vi "反馈节点 3.vi"() -> ()   [LabVIEW 2023]
panel:
  out "i=":i32
  out "x+1":dbl
  out "Array":dbl[](array[numeric])
  # "反馈节点 3"
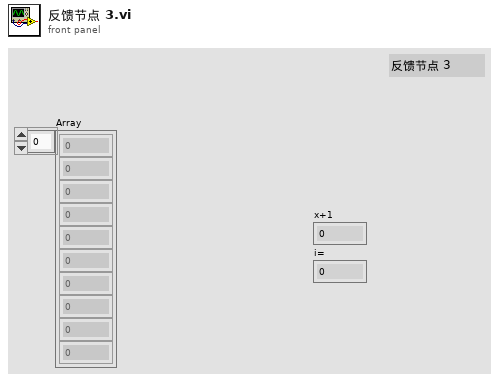
[diagram p1: front panel]
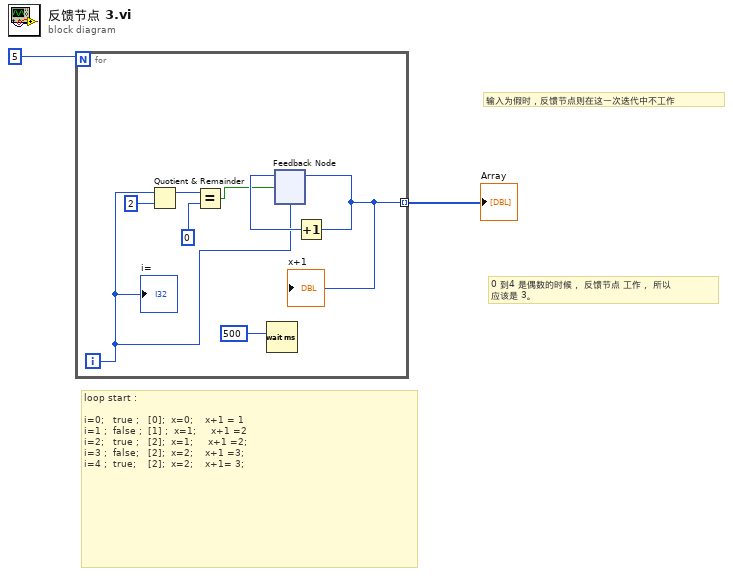
[diagram p0: block diagram]
diagram:
  # "0 到4 是偶数的时候， 反馈节点 工作， 所以 \n应该是 3。"
  # "loop start :\n\ni=0;   true ;   [0];  x=0;    x+1 = 1\ni=1 ;  false ;  [1] ;  x=1;     x+1 =2\ni=2;   true ;   [2];  x=1;     x+1 =2;\ni=3 ;  false;   [2];  x=2;    x+1 =3;\ni=4 ;  true;    [2];  x=2;    x+1= 3;"
  # "输入为假时，反馈节点则在这一次迭代中不工作"
  n1 = for {
    N: 5 -> [_]
    tunnel: [w4] -> w1 mode=indexing
    i -> [w3]
    n2 = Quotient & Remainder(x=w3, y=2) -> (x-y*floor(x/y)=w8:i32)  [unwired: 1 out]
    n3 = Equal?(x=w8, y=0) -> (x = y?=w6:bool)
    n4 = Wait (ms)(milliseconds to wait=500) -> ()  [unwired: 1 out]
    n5 = feedback #1(w3) -> (w10:i32)
    n6 = Increment(x=w10) -> (x+1=w4:i32)
    "x+1" <- w4
    n7 = feedback-in #1(w4, w6) -> ()
    "i=" <- w3
  }
  "Array" <- w1
